vi "WebDAV_Put_Files.vi"   [LabVIEW 2014]
uses:
  <vilib>/WebDAVClient/Simple Put File.vi
  <vilib>/WebDAVClient/NI_WebDAV.lvlib
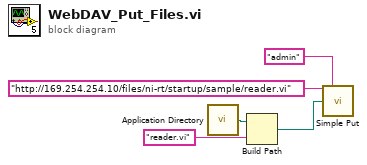
[diagram p0: block diagram]
diagram:
  n1 = call <vilib>:"Application Directory.vi"() -> ("Application Directory"=w4:path)
  n2 = Build Path(base path=w4, name or relative path="reader.vi") -> (appended path=w2:path)
  n3 = call-poly <vilib>:"Simple Put.vi"("file uri"="http://169.254.254.10/files/ni-rt/startup/sample/reader.vi" ("remote file uri"), "username"="admin", "local file path"=w2) -> ()  [unwired: 11 in, 2 out]
